vi "Ex. 2. Take a Voltage Measurement.vi"() -> ()   [LabVIEW 2024]
uses:
  <vilib>/measure/maspectr.llb/FFT Power Spectrum and PSD for N Chan.vi
  <vilib>/measure/NI_MAPro.lvlib
panel:
  in  "File Path":path
  out "Frequency-Domain Signal":cluster{"f0":dbl, "df":dbl, "magnitude":dbl[]}[](graph)
  in  "Stop":bool
  out "Time-Domain Signal":dynamicdata(graph)
  in  "Acquisition Rate":dbl(knob) scale=20000.0..30000.0
  # "Take a Voltage Measurement"
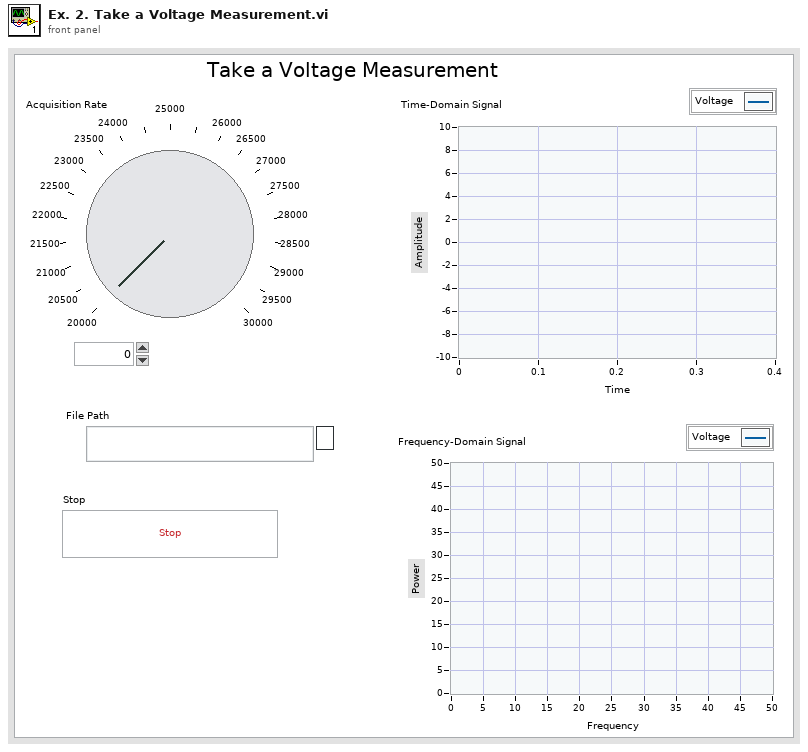
[diagram p1: front panel]
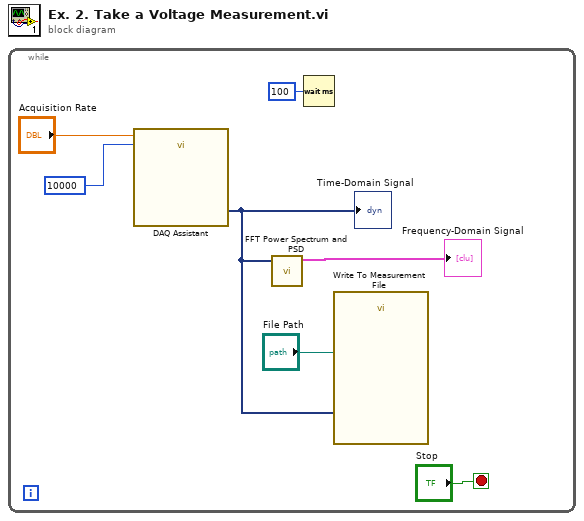
[diagram p0: block diagram]
diagram:
  n1 = while {
    stop <- "Stop" stop-if-true
    n2 = call "DAQ Assistant"("rate"="Acquisition Rate", "number of samples"=10000) -> ("data"=w2:dynamicdata)  [unwired: 15 in, 2 out]
    "Time-Domain Signal" <- w2
    n3 = call-poly <vilib>:"FFT Power Spectrum and PSD.vi"("time signals"=w2) -> ("Power Spectrum / PSD"=→"Frequency-Domain Signal":cluster{"f0":dbl, "df":dbl, "magnitude":dbl[]}[])  [unwired: 7 in, 3 out]
    n4 = Wait (ms)(milliseconds to wait=u32 100) -> ()  [unwired: 1 out]
    n5 = call "Write To Measurement File"("Signals"=w2, "Filename"="File Path") -> ()  [unwired: 15 in, 3 out]
  }
